vi "Volume entry-Event handler-Proceed.vi"(11 "ROI Info":T1 {"Zoom" min=1.0 max=10.0 step=0.10000000149011612}) -> (2 "Zoom":dbl, 3 "ROI Info []":T1[](array[typedef]) {"Zoom" min=1.0 max=10.0 step=0.10000000149011612})   [LabVIEW 2013]
uses:
  Typedefs/ROI spec.ctl
  Typedefs/ROI ID Enum.ctl
  ROI Entry screen/Globals/gl_Volume Entry UI globals.vi
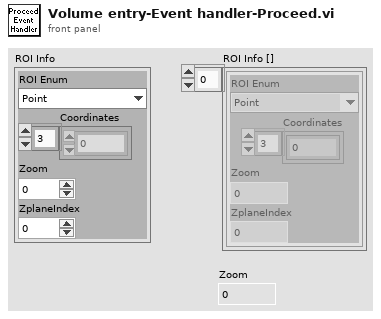
[diagram p1: front panel]
types:
  T1 = typedef "ROI spec.ctl" = cluster{"Coordinates":i32[], "Zoom":dbl, "ROI Enum":T2, "ZplaneIndex":i32}
  T2 = typedef "ROI ID Enum.ctl" = enum16{"Point", "MiniScan", "Comp. MiniScan", "Rectangle", "Comp. volume", "Arb. plane point"}
  T3 = typedef "Volume entry ctrl refs cluster.ctl" = cluster{"Z-step (planes)":refnum<vi>, "Volume":refnum<vi>, "Dual Rectangle":refnum<vi>, "Zoom":refnum<vi>, "Z-plane 1":refnum<vi>, "Z-plane 2":refnum<vi>, "ZplaneIndex (zero based)":refnum<vi>}
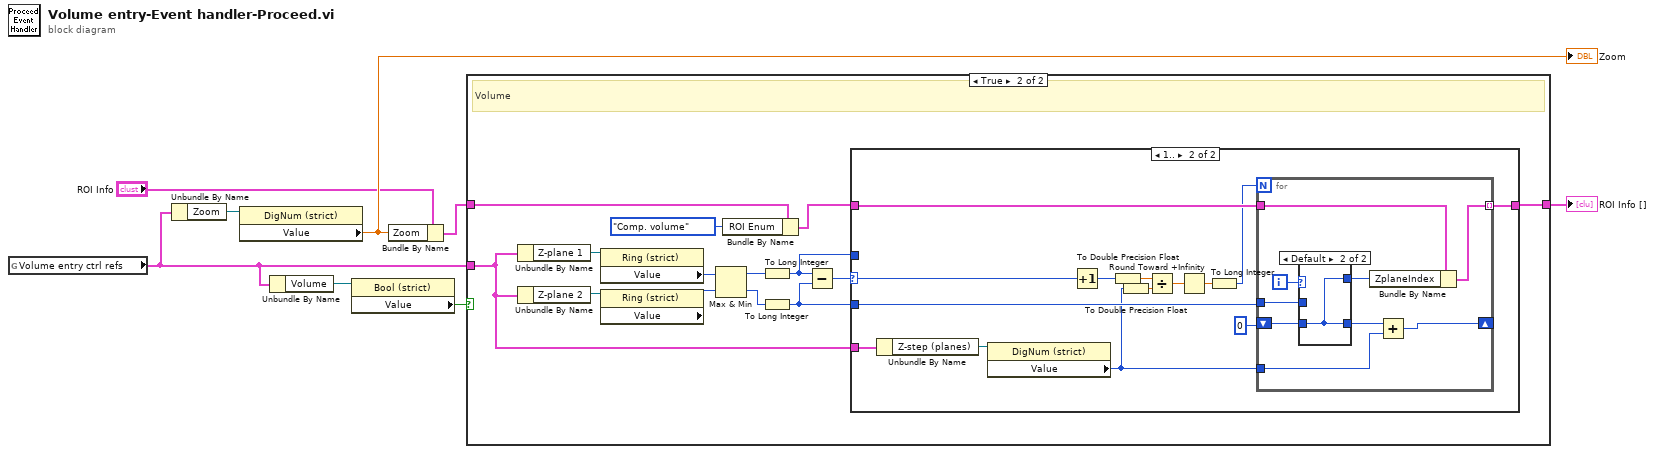
[diagram p0: block diagram]
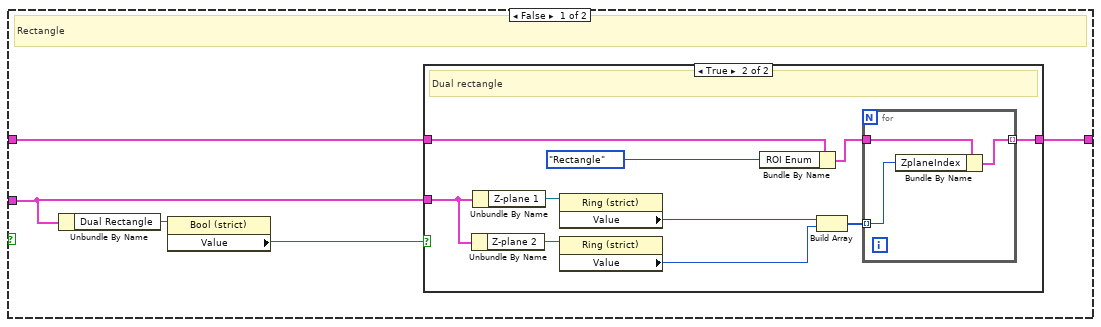
[diagram p2: hidden frame]
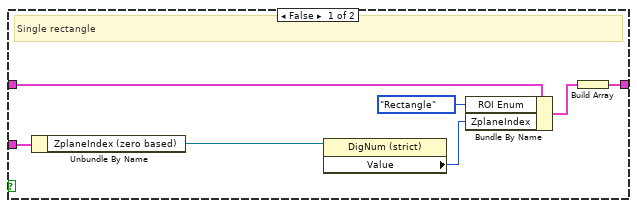
[diagram p3: hidden frame]
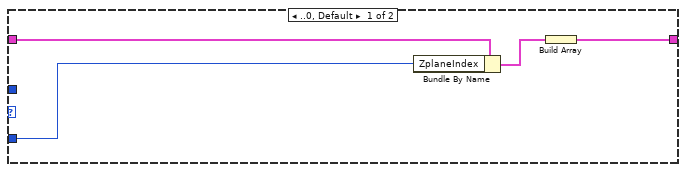
[diagram p4: hidden frame]
diagram:
  n1 = global read "gl_Volume Entry UI globals.vi" "Volume entry ctrl refs"() -> (w1:T3)
  n2 = Unbundle By Name(w1) -> ("Zoom"=w5:refnum<vi>)
  n3 = property on="Property Node" class="DigNum (strict)"(reference=w5) -> ("Value"=w6:dbl)  [unwired: 1 in, 2 out]
  "Zoom" <- w6
  n4 = Unbundle By Name(w1) -> ("Volume"=w7:refnum<vi>)
  n5 = property on="Property Node" class="Bool (strict)"(reference=w7) -> ("Value"=w8:bool)  [unwired: 1 in, 2 out]
  n6 = Bundle By Name(cluster="ROI Info", "Zoom"=w6) -> (w4:T1)
  n7 = case shown="True" w8 {
    tunnel: w4 -> [w12 w41]
    tunnel: [w13 w43] -> w2
    tunnel: w1 -> [w9 w34]
    frame False {
      # "Rectangle"
      n8 = Unbundle By Name(w9) -> ("Dual Rectangle"=w11:refnum<vi>)
      n9 = property class="Bool (strict)"(reference=w11) -> ("Value"=w10:bool)  [unwired: 1 in, 2 out]
      n10 = case shown="True" w10 {
        tunnel: [w20 w26] -> w13
        tunnel: w12 -> [w19 w27]
        tunnel: w9 -> [w14 w25]
        frame False {
          # "Single rectangle"
          n11 = Unbundle By Name(w14) -> ("ZplaneIndex (zero based)"=w16:refnum<vi>)
          n12 = property on="Property Node" class="DigNum (strict)"(reference=w16) -> ("Value"=w15:i32)  [unwired: 1 in, 2 out]
          n13 = Bundle By Name(cluster=w19, "ROI Enum"=ROI_ID_Enum."Rectangle", "ZplaneIndex"=w15) -> (w18:T1)
          n14 = Build Array(w18) -> (w20:T1[])
        }
        frame True {
          # "Dual rectangle"
          n15 = Unbundle By Name(w25) -> ("Z-plane 2"=w22:refnum<vi>)
          n16 = Unbundle By Name(w25) -> ("Z-plane 1"=w21:refnum<vi>)
          n17 = property class="Ring (strict)"(reference=w21) -> ("Value"=w24:u16)  [unwired: 1 in, 2 out]
          n18 = property class="Ring (strict)"(reference=w22) -> ("Value"=w23:u16)  [unwired: 1 in, 2 out]
          n19 = Bundle By Name(cluster=w27, "ROI Enum"=ROI_ID_Enum."Rectangle") -> (w29:T1)
          n20 = Build Array(w24, w23) -> (w30:u16[])
          n21 = for {
            tunnel: w29 -> [w33]
            tunnel: w30 -> [w32] mode=indexing
            tunnel: [w31] -> w26 mode=indexing
            n22 = Bundle By Name(cluster=w33, "ZplaneIndex"=w32) -> (w31:T1)
          }
        }
      }
    }
    frame True {
      # "Volume"
      n23 = Unbundle By Name(w34) -> ("Z-plane 1"=w38:refnum<vi>)
      n24 = Unbundle By Name(w34) -> ("Z-plane 2"=w37:refnum<vi>)
      n25 = property class="Ring (strict)"(reference=w38) -> ("Value"=w36:u16)  [unwired: 1 in, 2 out]
      n26 = property class="Ring (strict)"(reference=w37) -> ("Value"=w35:u16)  [unwired: 1 in, 2 out]
      n27 = Max & Min(x=w36, y=w35) -> (max(x,y)=w47:u16, min(x,y)=w46:u16)
      n28 = Bundle By Name(cluster=w41, "ROI Enum"=ROI_ID_Enum."Comp. volume") -> (w40:T1)
      n29 = To Long Integer(number=w47) -> (32bit integer=w45:i32)
      n30 = To Long Integer(number=w46) -> (32bit integer=w44:i32)
      n31 = Subtract(x=w45, y=w44) -> (x-y=w39:i32)
      n32 = case shown="1.." w39 {
        selector: w39 -> [_ w65]
        tunnel: w45 -> [_ _]
        tunnel: w44 -> [w48 w64]
        tunnel: w40 -> [w50 w62]
        tunnel: [w51 w61] -> w43
        tunnel: w34 -> [_ w54]
        frame ..0, Default {
          n33 = Bundle By Name(cluster=w50, "ZplaneIndex"=w48) -> (w49:T1)
          n34 = Build Array(w49) -> (w51:T1[])
        }
        frame 1.. {
          n35 = Unbundle By Name(w54) -> ("Z-step (planes)"=w56:refnum<vi>)
          n36 = property class="DigNum (strict)"(reference=w56) -> ("Value"=w55:i32)  [unwired: 1 in, 2 out]
          n37 = Increment(x=w65) -> (x+1=w60:i32)
          n38 = To Double Precision Float(number=w60) -> (double precision float=w53:dbl)
          n39 = To Double Precision Float(number=w55) -> (double precision float=w52:dbl)
          n40 = Divide(x=w53, y=w52) -> (x/y=w59:dbl)
          n41 = Round Toward +Infinity(x=w59) -> (ceil(x): smallest int >= x=w58:dbl)
          n42 = To Long Integer(number=w58) -> (32bit integer=w57:i32)
          n43 = for {
            N: w57 -> [_]
            tunnel: w64 -> [w73]
            shift-right: [w67] -> _
            shift-left: 0 -> [w72]
            tunnel: w62 -> [w71]
            tunnel: [w70] -> w61 mode=indexing
            tunnel: w55 -> [w66]
            i -> [w74]
            n44 = case shown="Default" w74 {
              tunnel: w73 -> [w75 _]
              tunnel: [w75 w76] -> w69
              tunnel: [w75 w76] -> w68
              tunnel: w72 -> [_ w76]
              frame 0 {
              }
              frame Default {
              }
            }
            n45 = Bundle By Name(cluster=w71, "ZplaneIndex"=w69) -> (w70:T1)
            n46 = Add(x=w68, y=w66) -> (x+y=w67:i32)
          }
        }
      }
    }
  }
  "ROI Info []" <- w2
